vi "Test3 Protocol Verification.vi"(8 "error in":errorcluster, 10 "CAN Frame Data":path=path "C:/Users/jlee/Documents/LabVIEW Projects/Tesla Assessment/Verification Product/test3.bin", 11 "Sequence Context In":refnum<k7>) -> (0 "error out":errorcluster={"status"=TRUE, "code"=7, "source"="Open/Create/Replace File in Test3 Protocol Verification.vi<APPEND>\nC:\\Users\\jlee\\Documents\\LabVIEW Projects\\Tesla Assessment\\Simple\\test3.bin"}, 3 "Values":sgl[](array[numeric]))   [LabVIEW 2021]
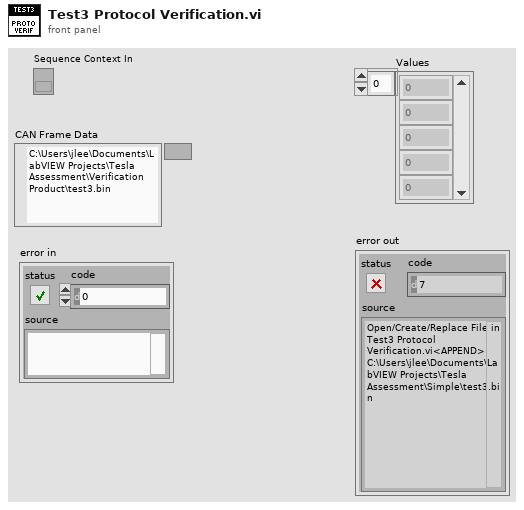
[diagram p1: front panel]
types:
  T1 = enum16{"big-endian, network order", "native, host order", "little-endian"}
  T2 = enum16{"open", "replace", "create", "open or create", "replace or create", "replace or create with confirmation"}
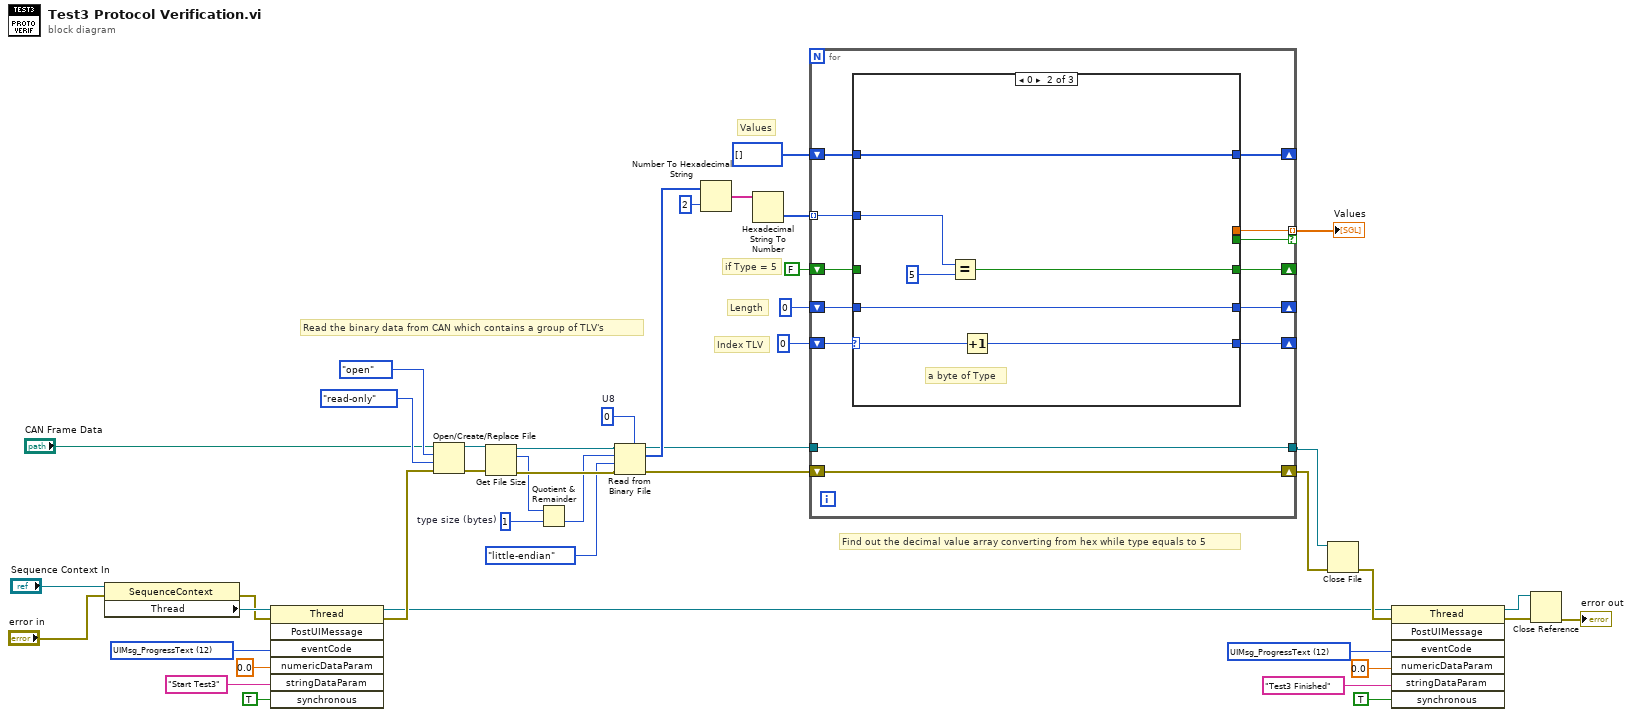
[diagram p0: block diagram]
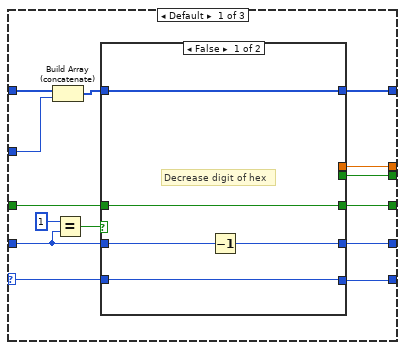
[diagram p2: hidden frame]
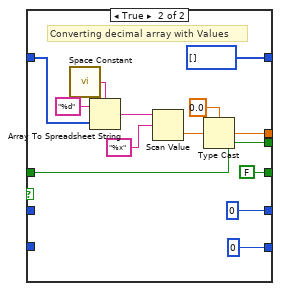
[diagram p3: hidden frame]
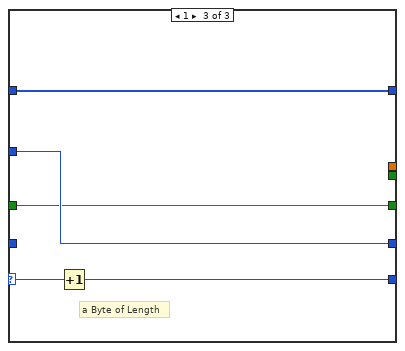
[diagram p4: hidden frame]
diagram:
  w10 = 12 items=["UIMsg_BreakOnUserRequest"=1, "UIMsg_BreakOnBreakpoint"=2, "UIMsg_BreakOnRunTimeError"=3, "UIMsg_Trace"=4, "UIMsg_TerminatingExecution"=5, "UIMsg_AbortingExecution"=6, "UIMsg_KillingExecutionThreads"=7, "UIMsg_EndExecution"=8, "UIMsg_ShutDownComplete"=9, "UIMsg_StartExecution"=10, "UIMsg_ProgressPercent"=11, "UIMsg_ProgressText"=12, "UIMsg_StartInteractiveExecution"=13, "UIMsg_EndInteractiveExecution"=14, "UIMsg_TerminatingInteractiveExecution"=15, "UIMsg_TerminationCancelled"=16, "UIMsg_ResumeFromBreak"=17, "UIMsg_StartFileExecution"=18, "UIMsg_EndFileExecution"=19, "UIMsg_ShutDownCancelled"=20, "UIMsg_LocalizationSettingChanged"=21, "UIMsg_OpenWindows"=22, "UIMsg_TileWindows"=23, "UIMsg_CascadeWindows"=24, "UIMsg_ReportChanged"=25, "UIMsg_CloseWindows"=26, "UIMsg_RefreshWindows"=27, "UIMsg_ClientFileChanged"=28, "UIMsg_DisplayReport"=29, "UIMsg_ModelState_Initializing"=30, "UIMsg_ModelState_Waiting"=31, "UIMsg_ModelState_Identified"=32, "UIMsg_ModelState_BeginTesting"=33, "UIMsg_ModelState_TestingComplete"=34, "UIMsg_ModelState_PostProcessingComplete"=35, "UIMsg_ModelState_EnabledStateSet"=36, "UIMsg_ReportLocationChanged"=37, "UIMsg_GotoLocation"=38, "UIMsg_PushUndoItem"=39, "UIMsg_OutputMessages"=40, "UIMsg_TypePaletteFileListChanged"=41, "UIMsg_NonTerminatableThreadsArePreventingTermination"=42, "UIMsg_ModelState_PostProcessing"=43, "UIMsg_ReportCollectionChanged"=44, "UIMsg_RuntimeError"=45, "UIMsg_UserMessageBase"=10000] ("eventCode")
  w17 = 12 items=["UIMsg_BreakOnUserRequest"=1, "UIMsg_BreakOnBreakpoint"=2, "UIMsg_BreakOnRunTimeError"=3, "UIMsg_Trace"=4, "UIMsg_TerminatingExecution"=5, "UIMsg_AbortingExecution"=6, "UIMsg_KillingExecutionThreads"=7, "UIMsg_EndExecution"=8, "UIMsg_ShutDownComplete"=9, "UIMsg_StartExecution"=10, "UIMsg_ProgressPercent"=11, "UIMsg_ProgressText"=12, "UIMsg_StartInteractiveExecution"=13, "UIMsg_EndInteractiveExecution"=14, "UIMsg_TerminatingInteractiveExecution"=15, "UIMsg_TerminationCancelled"=16, "UIMsg_ResumeFromBreak"=17, "UIMsg_StartFileExecution"=18, "UIMsg_EndFileExecution"=19, "UIMsg_ShutDownCancelled"=20, "UIMsg_LocalizationSettingChanged"=21, "UIMsg_OpenWindows"=22, "UIMsg_TileWindows"=23, "UIMsg_CascadeWindows"=24, "UIMsg_ReportChanged"=25, "UIMsg_CloseWindows"=26, "UIMsg_RefreshWindows"=27, "UIMsg_ClientFileChanged"=28, "UIMsg_DisplayReport"=29, "UIMsg_ModelState_Initializing"=30, "UIMsg_ModelState_Waiting"=31, "UIMsg_ModelState_Identified"=32, "UIMsg_ModelState_BeginTesting"=33, "UIMsg_ModelState_TestingComplete"=34, "UIMsg_ModelState_PostProcessingComplete"=35, "UIMsg_ModelState_EnabledStateSet"=36, "UIMsg_ReportLocationChanged"=37, "UIMsg_GotoLocation"=38, "UIMsg_PushUndoItem"=39, "UIMsg_OutputMessages"=40, "UIMsg_TypePaletteFileListChanged"=41, "UIMsg_NonTerminatableThreadsArePreventingTermination"=42, "UIMsg_ModelState_PostProcessing"=43, "UIMsg_ReportCollectionChanged"=44, "UIMsg_RuntimeError"=45, "UIMsg_UserMessageBase"=10000] ("eventCode")
  w32 = u8 0  # U8
  w39 = i64 1  # type size (bytes)
  # "Find out the decimal value array converting from hex while type equals to 5"
  # "Read the binary data from CAN which contains a group of TLV's"
  # "if Type = 5"
  # "Values"
  # "Length"
  # "Index TLV"
  n1 = property class="SequenceContext"(reference="Sequence Context In", error in="error in") -> (error out=w15:errorcluster, "Thread"=w16:refnum<k7>)  [unwired: 1 out]
  n2 = invoke class="Thread" method="PostUIMessage"(reference=w16, error in=w15, "eventCode"=w17, "numericDataParam"=0.0, "stringDataParam"="Start Test3", "synchronous"=TRUE) -> (reference out=w8:refnum<k7>, error out=w14:errorcluster)  [unwired: 1 in, 5 out]
  n3 = Open/Create/Replace File(file path (use dialog)="CAN Frame Data", error in=w14, operation (0:open)=T2."open", access (0:read/write)=enum16{"read/write", "read-only", "write-only"}."read-only") -> (refnum out=w41:refnum<file>, error out=w40:errorcluster)  [unwired: 2 in, 1 out]
  n4 = Get File Size(file=w41, error in=w40) -> (refnum out=w37:refnum<file>, size (in bytes)=w35:i64, 0:w38:errorcluster)
  n5 = Quotient & Remainder(x=w35, y=w39) -> (floor(x/y)=w31:i64)  [unwired: 1 out]
  n6 = Read from Binary File(5:w32, 8:w38, 9:T1."little-endian" ("byte order (0:big-endian, network order)"), 10:w31, 11:w37) -> (0:w4:errorcluster, 2:w33:u8[], 3:w3:refnum<file>)  [unwired: 1 in, 1 out]
  n7 = Number To Hexadecimal String(1:i16 2 ("width (-)"), 2:w33) -> (0:w30:string[])
  n8 = Hexadecimal String To Number(string=w30) -> (number=w29:u32[])  [unwired: 2 in, 1 out]
  n9 = for {
    tunnel: w29 -> [w55] mode=indexing
    shift-right: [w53] -> _
    shift-left: u32[] [] -> [w54]
    shift-right: [w50] -> _
    shift-left: u32 0 ("element") -> [w56]
    tunnel: [w49] -> w26 mode=indexing if=w46
    shift-right: [w51] -> _
    shift-left: u32 0 ("element") -> [w52]
    shift-right: [w48] -> _
    shift-left: FALSE -> [w47]
    tunnel: [w44] -> w1
    tunnel: w3 -> [w44]
    shift-right: [w45] -> w2
    shift-left: w4 -> [w45]
    n10 = case shown="0" w56 {
      selector: w56 -> [w60 w95 w100]
      tunnel: [w67 w93 w97] -> w50
      tunnel: w55 -> [w62 w90 w99]
      tunnel: w54 -> [w63 w94 w98]
      tunnel: [w70 w94 w98] -> w53
      tunnel: w52 -> [w65 w92 _]
      tunnel: [w69 w92 w99] -> w51
      tunnel: [w68 _ _] -> w49
      tunnel: [w58 w91 w96] -> w48
      tunnel: w47 -> [w59 _ w96]
      tunnel: [w57 _ _] -> w46
      frame Default {
        # "Not 0 and 1"
        n11 = Build Array (concatenate)(w63, w62) -> (w61:u32[])
        n12 = Equal?(x=u32 1 ("y"), y=w65) -> (x = y?=w64:bool)
        n13 = case shown="False" w64 {
          tunnel: [w73 u32[] []] -> w70
          tunnel: w65 -> [w75 _]
          tunnel: [w74 u32 0] -> w69
          tunnel: [_ w81] -> w68
          tunnel: [w72 u32 0] -> w67
          tunnel: w61 -> [w73 w78]
          tunnel: w60 -> [w72 _]
          tunnel: w59 -> [w71 w77]
          tunnel: [w71 FALSE] -> w58
          tunnel: [_ w77] -> w57
          frame False {
            # "Decrease digit of hex"
            n14 = Decrement(x=w75) -> (x-1=w74:u32)
          }
          frame True {
            # "Converting decimal array with Values"
            n15 = call <vilib>:"Space Constant.vi"() -> ("String"=w86:string)
            n16 = Array To Spreadsheet String(delimiter (Tab)=w86, array=w78, 3:"%d" ("format string")) -> (spreadsheet string=w87:string)
            n17 = Scan Value(string=w87, format string="%x") -> (value=w85:dbl)  [unwired: 1 in, 1 out]
            n18 = Type Cast(type=sgl 0.0, x=w85) -> (*(type *) &x=w81:sgl)
          }
        }
      }
      frame 0 {
        # "a byte of Type"
        n19 = Equal?(x=w90, y=u32 5 ("element")) -> (x = y?=w91:bool)
        n20 = Increment(x=w95) -> (x+1=w93:u32)
      }
      frame 1 {
        # "a Byte of Length"
        n21 = Increment(x=w100) -> (x+1=w97:u32)
      }
    }
  }
  "Values" <- w26
  n22 = Close File(refnum=w1, error in=w2) -> (error out=w9:errorcluster)  [unwired: 1 out]
  n23 = invoke class="Thread" method="PostUIMessage"(reference=w8, error in=w9, "eventCode"=w10, "numericDataParam"=0.0, "stringDataParam"="Test3 Finished", "synchronous"=TRUE) -> (reference out=w5:refnum<k7>, error out=w7:errorcluster)  [unwired: 1 in, 5 out]
  n24 = Close Reference(reference=w5, error in (no error)=w7) -> (error out=→"error out":errorcluster)
